vi "Sett_UP_Convert.vi"(8 "error in (no error)":errorcluster, 9 "Divider":dbl, 11 "RFID system in":refnum<class "RFID system.lvclass">) -> (0 "error out":errorcluster, 2 "Waveform":waveform(dbl), 3 "RFID system out":refnum<class "RFID system.lvclass">)   [LabVIEW 2019, in "RFID system.lvclass"]
uses:
  RFID system.lvclass
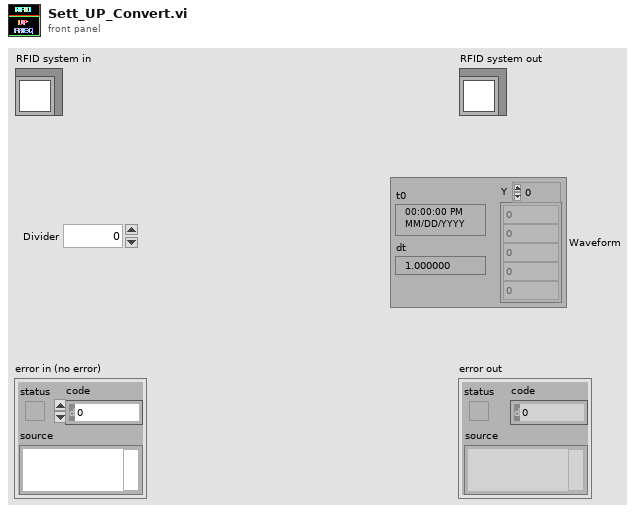
[diagram p1: front panel]
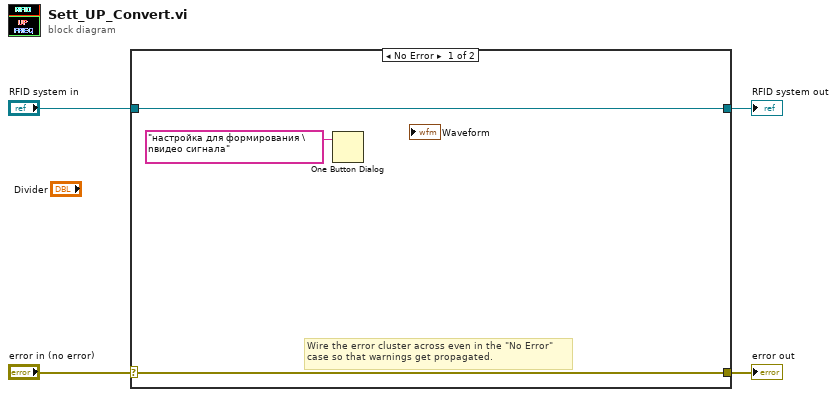
[diagram p0: block diagram]
diagram:
  n1 = case shown="No Error" "error in (no error)" {
    selector: "error in (no error)" -> [w6 w9]
    tunnel: [w6 w9] -> w3
    tunnel: [w7 w8] -> w1
    tunnel: "RFID system in" -> [w7 w8]
    frame No Error {
      # "Wire the error cluster across even in the \"No Error\"\ncase so that warnings get propagated."
      n2 = One Button Dialog(message="настройка для формирования \nвидео сигнала") -> ()  [unwired: 1 in, 1 out]
    }
    frame Error {
    }
  }
  "error out" <- w3
  "RFID system out" <- w1
